vi "emi_FP Origin top left.vi"(5 "VI Refnum(This vi)":refnum<vi>, 9 "error in (no error)":errorcluster, 12 "All panes(T)":bool=TRUE) -> (6 "VI Refnum":refnum<vi>, 10 "error out":errorcluster)   [LabVIEW 2011]
doc: "Places the front panel origin (0,0) to top left of visible window.\n\nIf no VI ref in, then the VI containing this VI is used.\nIf VI has multiple panes, only the first pane will be used.\n\nOn error in: Does not run."
uses:
  <vilib>/Utility/miscctls.llb/LVPointTypeDef.ctl
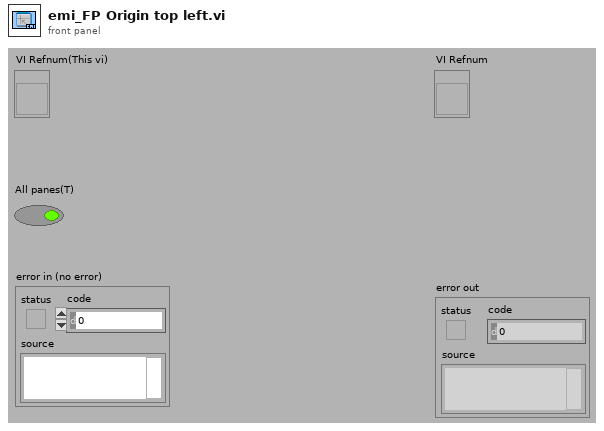
[diagram p1: front panel]
types:
  T1 = typedef "LVPointTypeDef.ctl" = cluster{"Horizontal":i16, "Vertical":i16}
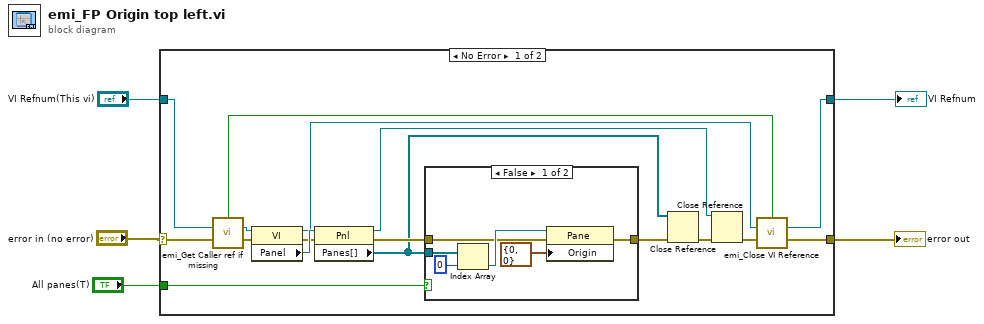
[diagram p0: block diagram]
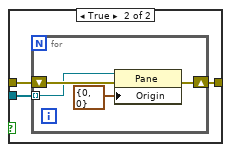
[diagram p2: hidden frame]
diagram:
  n1 = case shown="No Error" "error in (no error)" {
    selector: "error in (no error)" -> [w15 w37]
    tunnel: [w9 w37] -> w5
    tunnel: "VI Refnum(This vi)" -> [w14 w36]
    tunnel: [w8 w36] -> w3
    tunnel: "All panes(T)" -> [w6 _]
    frame No Error {
      n2 = call "emi_Get Caller ref if missing.vi"("VI Refnum(Calling VI)"=w14, "error in (no error)"=w15) -> ("Ref Generated"=w16:bool, "VI Refnum Out"=w12:refnum<vi>, "error out"=w13:errorcluster)  [unwired: 11 in]
      n3 = property class="VI"(reference=w12, error in=w13) -> (reference out=w11:refnum<vi>, error out=w21:errorcluster, "Panel"=w22:refnum<vi>)
      n4 = property class="Pnl"(reference=w22, error in=w21) -> (reference out=w17:refnum<vi>, error out=w20:errorcluster, "Panes[]"=w7:refnum<vi>[])
      n5 = case shown="False" w6 {
        tunnel: w20 -> [w26 w31]
        tunnel: [w24 w30] -> w19
        tunnel: w7 -> [w23 w29]
        frame False {
          n6 = Index Array(array=w23, index=0) -> (element=w27:refnum<vi>)
          n7 = property class="Pane"(reference=w27, error in=w26, "Origin"=T1 {"Horizontal"=0, "Vertical"=0}) -> (error out=w24:errorcluster)  [unwired: 1 out]
        }
        frame True {
          n8 = for {
            tunnel: w29 -> [w32] mode=indexing
            shift-right: [w33] -> w30
            shift-left: w31 -> [w35]
            n9 = property class="Pane"(reference=w32, error in=w35, "Origin"=T1 {"Horizontal"=0, "Vertical"=0}) -> (error out=w33:errorcluster)  [unwired: 1 out]
          }
        }
      }
      n10 = Close Reference(reference=w7, error in (no error)=w19) -> (error out=w18:errorcluster)
      n11 = Close Reference(reference=w17, error in (no error)=w18) -> (error out=w10:errorcluster)
      n12 = call "emi_Close VI Reference.vi"("Close ref?(T)"=w16, "VI Refnum"=w11, "error in (no error)"=w10) -> ("VI Refnum Out"=w8:refnum<vi>, "error out"=w9:errorcluster)  [unwired: 11 in]
    }
    frame Error {
    }
  }
  "error out" <- w5
  "VI Refnum" <- w3
